vi "img2ByteArr.vi"(6 "kwarg_name":string, 8 "error in (no error)":errorcluster, 11 "img in":T3) -> (0 "error out":errorcluster, 2 "Bindata & descr out":T1, 3 "flattened data out":u8[](array[numeric]))   [LabVIEW 2018, in "LV2Julia_core.lvlib"]
uses:
  LV2Julia_core.lvlib
  <vilib>/picture/picture.llb/imagedata.ctl
  Bindata&description.ctl
  Bindata description.ctl
  6302e4ae-4b40-419b-b28c-52cb7b14de06.vi
  6302e4ae-4b40-419b-b28c-52cb7b14de06.vi/fee58b07-59ca-4fa2-b889-50445a9ab99e.vi
  <vilib>/Utility/error.llb/Error Cluster From Error Code.vi
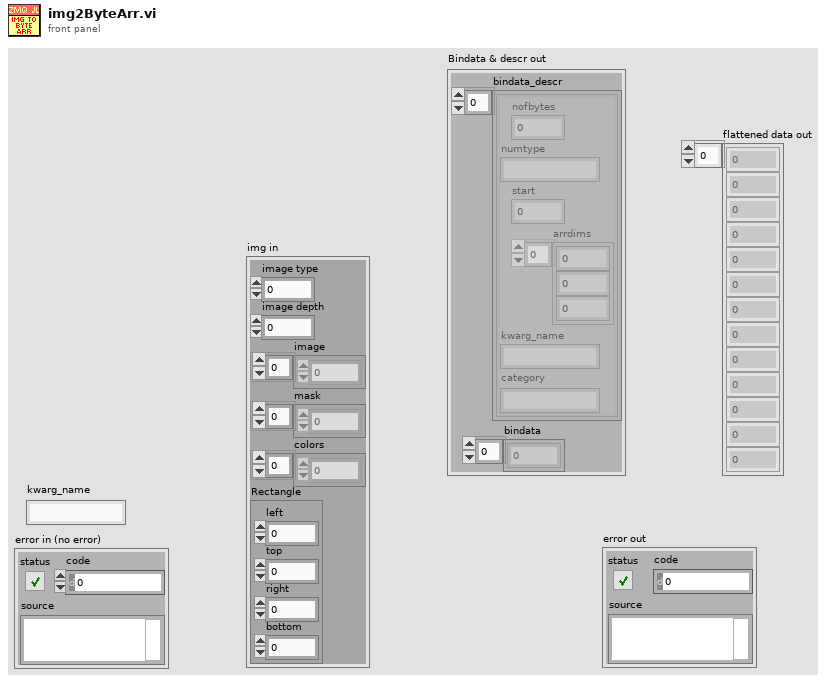
[diagram p1: front panel]
types:
  T1 = typedef "LV2Julia_core.lvlib/Bindata&description.ctl" = cluster{"bindata_descr":T2[], "bindata":u8[]}
  T2 = typedef "LV2Julia_core.lvlib/Bindata description.ctl" = cluster{"nofbytes":i32, "numtype":string, "start":i32, "arrdims":i32[], "kwarg_name":string, "category":string}
  T3 = typedef "imagedata.ctl" = cluster{"image type":i32, "image depth":i32, "image":u8[], "mask":u8[], "colors":u32[], "Rectangle":cluster{"left":i16, "top":i16, "right":i16, "bottom":i16}}
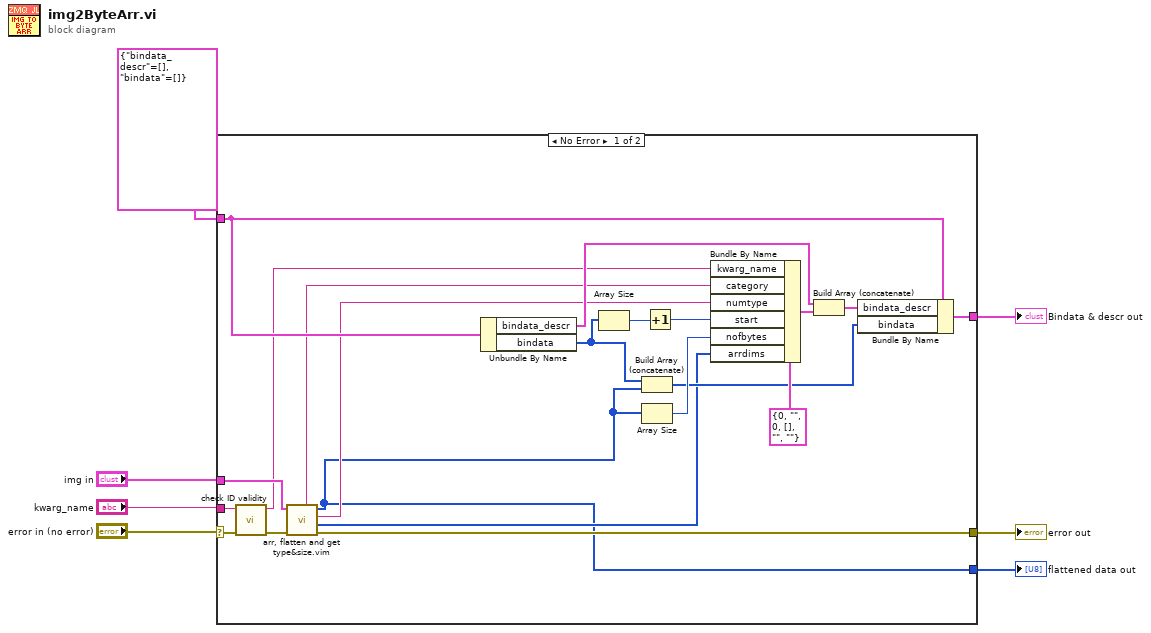
[diagram p0: block diagram]
diagram:
  n1 = case shown="No Error" "error in (no error)" {
    selector: "error in (no error)" -> [w23 w29]
    tunnel: "img in" -> [w24 _]
    tunnel: [w8 _] -> w6
    tunnel: "kwarg_name" -> [w22 _]
    tunnel: T1 {"bindata_descr"=[], "bindata"=[]} ("Bindata & descr in") -> [w21 _]
    tunnel: [w19 _] -> w2
    tunnel: [w14 w29] -> w1
    frame No Error {
      n2 = call "check ID validity.vi"("error in (no error)"=w23, "ID in"=w22) -> ("error out"=w13:errorcluster, "ID out"=w10:string)  [unwired: 8 in]
      n3 = call "arr, flatten and get type&size.vim"("error in (no error)"=w13, "data in"=w24) -> ("error out"=w14:errorcluster, "sizes"=w12:i16[], "numtype"=w11:string, "flattened array out"=w8:u8[], "category"=w9:string)  [unwired: 5 in]
      n4 = Unbundle By Name(w21) -> ("bindata_descr"=w17:T2[], "bindata"=w20:u8[])
      n5 = Array Size(array=w20) -> (size(s)=w28:i32)
      n6 = Build Array (concatenate)(w20, w8) -> (w18:u8[])
      n7 = Array Size(array=w8) -> (size(s)=w25:i32)
      n8 = Increment(x=w28) -> (x+1=w26:i32)
      n9 = Bundle By Name(cluster=T2 {"nofbytes"=0, "numtype"="", "start"=0, "arrdims"=[], "kwarg_name"="", "category"=""} ("bindata descr"), "kwarg_name"=w10, "category"=w9, "numtype"=w11, "start"=w26, "nofbytes"=w25, "arrdims"=w12) -> (w15:T2)
      n10 = Build Array (concatenate)(w17, w15) -> (w16:T2[])
      n11 = Bundle By Name(cluster=w21, "bindata_descr"=w16, "bindata"=w18) -> (w19:T1)
    }
    frame Error {
    }
  }
  "flattened data out" <- w6
  "error out" <- w1
  "Bindata & descr out" <- w2
